vi "EventLog.FormatErrorMessage.vi"(1 "Error string in":string) -> (0 "Error string out":string)   [LabVIEW 2016]
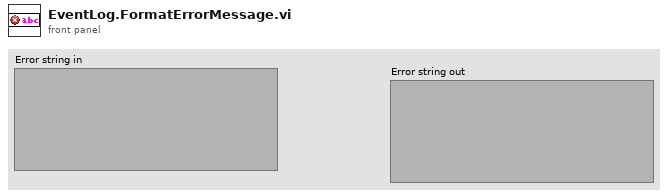
[diagram p1: front panel]
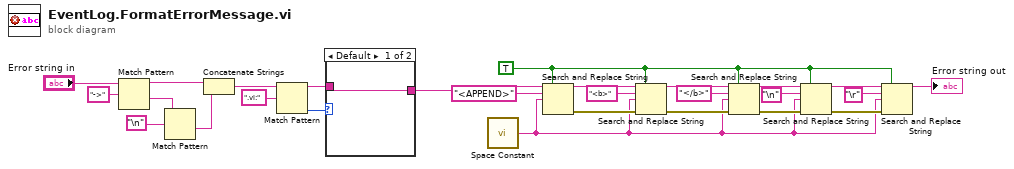
[diagram p0: block diagram]
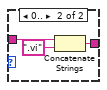
[diagram p2: hidden frame]
diagram:
  w8 = TRUE ("replace all? (F)")
  n1 = Match Pattern(string="Error string in", regular expression="->") -> (before substring=w23:string, after substring=w25:string)  [unwired: 1 in, 2 out]
  n2 = Match Pattern(string=w25, regular expression="\n") -> (after substring=w22:string)  [unwired: 1 in, 3 out]
  n3 = Concatenate Strings(w23, w22) -> (w6:string)
  n4 = Match Pattern(string=w6, regular expression=".vi:" ("search string")) -> (before substring=w5:string, offset past match=w2:i32)  [unwired: 1 in, 2 out]
  n5 = case shown="Default" w2 {
    tunnel: w5 -> [w28 w31]
    tunnel: [w28 w30] -> w3
    frame Default {
    }
    frame 0.. {
      n6 = Concatenate Strings(w31, ".vi" ("string")) -> (w30:string)
    }
  }
  n7 = call <vilib>:"Space Constant.vi"() -> ("String"=w7:string)
  n8 = Search and Replace String(replace all?=w8, input string=w3, search string="<APPEND>", replace string=w7) -> (result string=w20:string, error out=w14:errorcluster)  [unwired: 4 in, 2 out]
  n9 = Search and Replace String(replace all?=w8, input string=w20, search string="<b>", replace string=w7, error in=w14) -> (result string=w19:string, error out=w15:errorcluster)  [unwired: 3 in, 2 out]
  n10 = Search and Replace String(replace all?=w8, input string=w19, search string="</b>", replace string=w7, error in=w15) -> (result string=w16:string, error out=w17:errorcluster)  [unwired: 3 in, 2 out]
  n11 = Search and Replace String(replace all?=w8, input string=w16, search string="\n", replace string=w7, error in=w17) -> (result string=w11:string, error out=w10:errorcluster)  [unwired: 3 in, 2 out]
  n12 = Search and Replace String(replace all?=w8, input string=w11, search string="\r", replace string=w7, error in=w10) -> (result string=→"Error string out":string)  [unwired: 3 in, 3 out]
